vi "WaitForClosureOfSubVI.vi"(8 "error in (no error)":errorcluster, 11 "Controls Reference Out":T1) -> (0 "error out":errorcluster)   [LabVIEW 2015]
uses:
  AODControl/AODControlFiles/LoadControl.ctl
  AODControl/AODControl.lvlib
  AODControl/AODControlFiles/InterfaceReferences.ctl
  AODControl/AODControlFiles/ExitButton.ctl
  ImageAcquisitionProgram/ImageAcquisitionLibrary/InterfaceReferences.ctl
  ImageAcquisitionProgram/ImageAcquisitionLibrary.lvlib
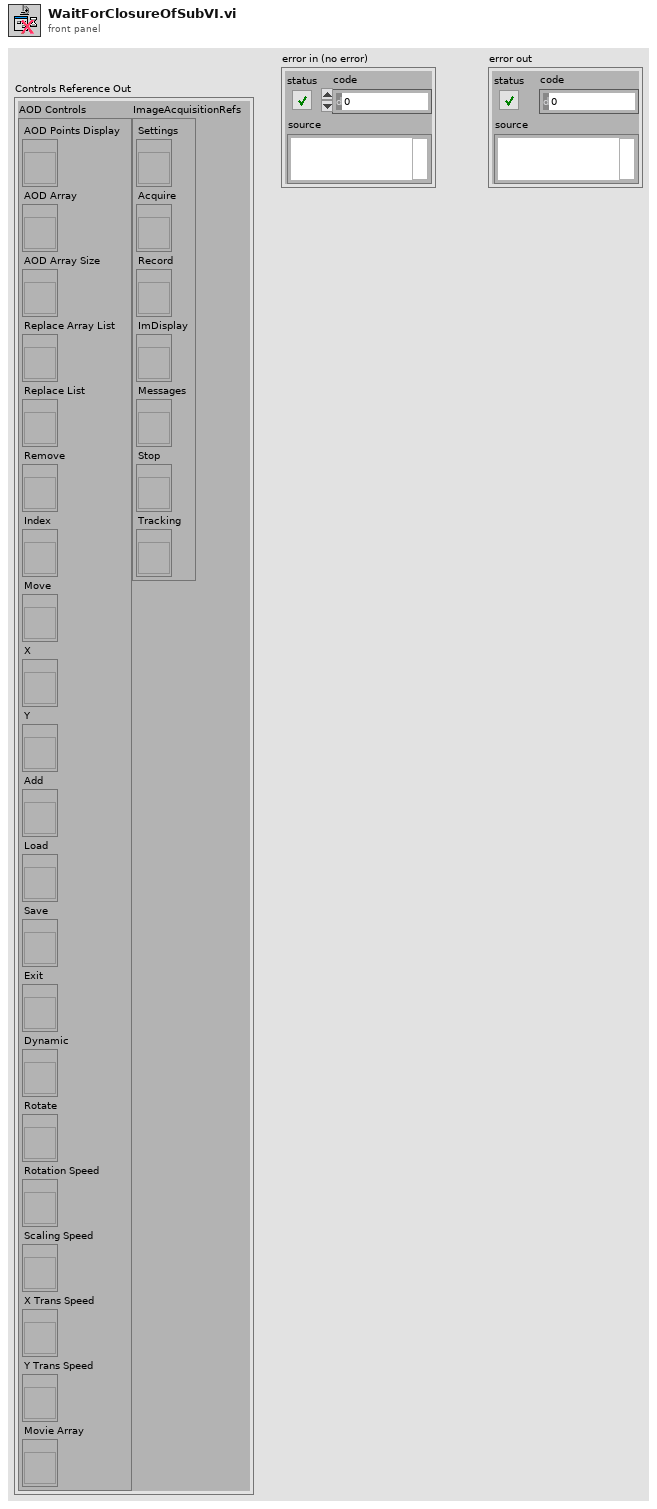
[diagram p1: front panel]
types:
  T1 = typedef "ExperimentControls" = cluster{"AOD Controls":T2, "ImageAcquisitionRefs":T3}
  T2 = typedef "AODControl.lvlib/InterfaceReferences.ctl" = cluster{"AOD Points Display":refnum<vi>, "AOD Array":refnum<vi>, "AOD Array Size":refnum<vi>, "Replace Array List":refnum<vi>, "Replace List":refnum<vi>, "Remove":refnum<vi>, "Index":refnum<vi>, "Move":refnum<vi>, "X":refnum<vi>, "Y":refnum<vi>, "Add":refnum<vi>, "Load":refnum<vi>, "Save":refnum<vi>, "Exit":refnum<vi>, "Dynamic":refnum<vi>, "Rotate":refnum<vi>, "Rotation Speed":refnum<vi>, "Scaling Speed":refnum<vi>, "X Trans Speed":refnum<vi>, "Y Trans Speed":refnum<vi>, "Movie Array":refnum<vi>}
  T3 = typedef "ImageAcquisitionLibrary.lvlib/InterfaceReferences.ctl" = cluster{"Settings":refnum<vi>, "Acquire":refnum<vi>, "Record":refnum<vi>, "ImDisplay":refnum<vi>, "Messages":refnum<vi>, "Stop":refnum<vi>, "Tracking":refnum<vi>}
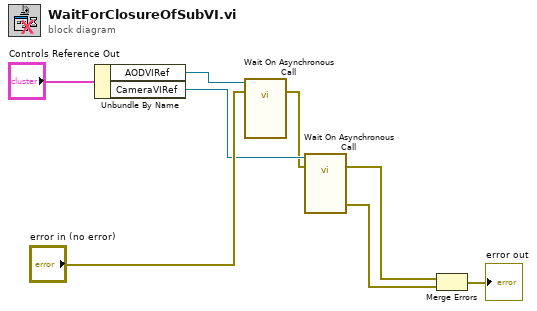
[diagram p0: block diagram]
diagram:
  n1 = Unbundle By Name("Controls Reference Out") -> ("AODVIRef"=w8:refnum<vi>, "CameraVIRef"=w5:refnum<vi>)
  n2 = call-by-ref "Wait On Asynchronous Call"(reference=w8, error in="error in (no error)") -> (error out=w1:errorcluster)  [unwired: 12 in, 1 out]
  n3 = call-by-ref "Wait On Asynchronous Call"(reference=w5, error in=w1) -> (error out=w3:errorcluster, 0:"error out"=w2:errorcluster)  [unwired: 11 in, 1 out]
  n4 = Merge Errors(w3, w2) -> (→"error out":errorcluster)
